vi "get prog command 3.vi"(0 "Data":u32) -> (1 "aux (24)":u32, 2 "command":T1(ring) format="%x")   [LabVIEW 2019]
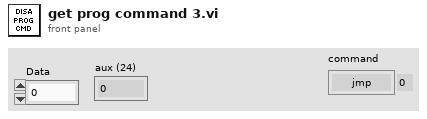
[diagram p1: front panel]
types:
  T1 = enum8{"jmp", "dly", "Con0 P0 out", "dds0 aux", "dds1 aux", "dds0 cmd", "dds1 cmd", "AOwfm", "AIacq", "rec ctl", "irq0", "dma point ", "stall", "dds2 aux", "dds3 aux", "dds2 cmd", "dds3 cmd", "trigwait", "jmp_X", "jmp_Y", "mcdA_init", "jmp_mcdA", "init_T", "jmp_T", "read_mcdA", "reset_jmp"}
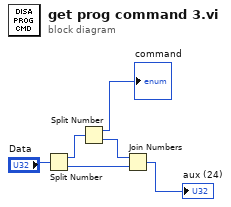
[diagram p0: block diagram]
diagram:
  n1 = Split Number(x="Data") -> (hi(x)=w3:u16, lo(x)=w5:u16)
  n2 = Split Number(x=w3) -> (hi(x)=→"command":u8, lo(x)=w4:u8)
  n3 = Join Numbers(hi=w4, lo=w5) -> ((hi.lo)=→"aux (24)":u32)
